vi "Get Buffer.vi"(8 "error in (no error)":errorcluster, 11 "Carya Config (Buffer) in":refnum<class "CConfig Nonpersistant Buffer.lvclass">) -> (0 "error out":errorcluster, 1 "Copy data?":bool=TRUE, 2 "Config":refnum<class "Carya Config.lvclass">, 3 "Carya Config (Buffer) out":refnum<class "CConfig Nonpersistant Buffer.lvclass">)   [LabVIEW 2013, in "CConfig Nonpersistant Buffer.lvclass"]
doc: "Copyright 2018, Carya Automatisering, Wiebe Walstra."
uses:
  CConfig Nonpersistant Buffer.lvclass
  Carya Config.lvclass
  CConfig Nonpersistant Buffer.lvclass/CConfig Nonpersistant Buffer.ctl
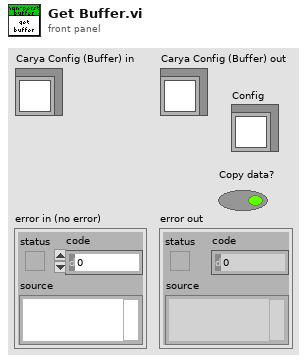
[diagram p1: front panel]
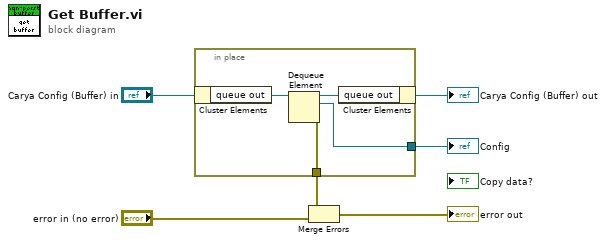
[diagram p0: block diagram]
diagram:
  n1 = in-place "In Place Element Structure" {
    in-place-border: [w8] -> w3
    in-place-border: [w7] -> w1
    n2 = in-place-cluster #1("Carya Config (Buffer) in") -> ("queue out"=w10:refnum<queue>)
    n3 = Dequeue Element(queue=w10) -> (queue out=w9:refnum<queue>, element=w8:refnum<class "Carya Config.lvclass">, error out=w7:errorcluster)  [unwired: 2 in, 1 out]
    n4 = in-place-cluster #1("queue out"=w9) -> (→"Carya Config (Buffer) out":refnum<class "CConfig Nonpersistant Buffer.lvclass">)
  }
  "Config" <- w3
  n5 = Merge Errors(w1, "error in (no error)") -> (→"error out":errorcluster)
